vi "example test.vi"() -> ()   [LabVIEW 2014, in "alarms module tests.lvlib"]
uses:
  alarms module tests.lvlib
  module/configuration/alarms module configuration.lvclass
  module/execution/alarms module runtime.lvclass
  module/configuration/alarm configuration.ctl
  module/configuration/alarm comparison.ctl
  <vilib>/NI/Tag Bus Module Framework/channel/TBM channel.lvclass
  module/configuration/compare type.ctl
  module/configuration/boolean operation.ctl
  <vilib>/NI/Tag Bus/tag/Data Type.ctl
  <vilib>/NI/Tag Bus Module Framework/channel/channel classification.ctl
  module/configuration/alarms module configuration.lvclass/alarms module configuration.ctl
  <vilib>/NI/Tag Bus/tag/tag descriptor.lvclass/tag descriptor.ctl
  <vilib>/NI/Tag Bus/table/data polymorphs/write one/write Boolean.vi
  <vilib>/NI/Tag Bus/table/data polymorphs/write one/write Double.vi
  <vilib>/NI/Tag Bus/table/data polymorphs/write one/write U64.vi
  <vilib>/NI/Tag Bus/table/data polymorphs/read one/read Boolean.vi
  module/configuration/Write alarms.vi
  <vilib>/NI/Tag Bus/tag/read tag name.vi
  <vilib>/NI/Tag Bus/dictionary/locate tag.vi
  <vilib>/NI/Configuration Framework/serializable configuration/NISE_CEF_serializable configuration.lvclass
  <vilib>/NI/Tag Bus/tag/tag descriptor.lvclass
  <vilib>/NI/Tag Bus/dictionary/data dictionary.lvclass
  <vilib>/NI/Tag Bus/table/data table.lvlib
panel:
  in  "a":dbl
  in  "b":u64
  in  "unlatch":bool
  in  "stop":bool
  out "out":bool
  out "final error":errorcluster
  out "output error":errorcluster
  out "input lookup error":errorcluster
  out "init error":errorcluster
  out "correct execution settings":bool
  out "serialization problem":errorcluster
  out "invalid configuration":errorcluster
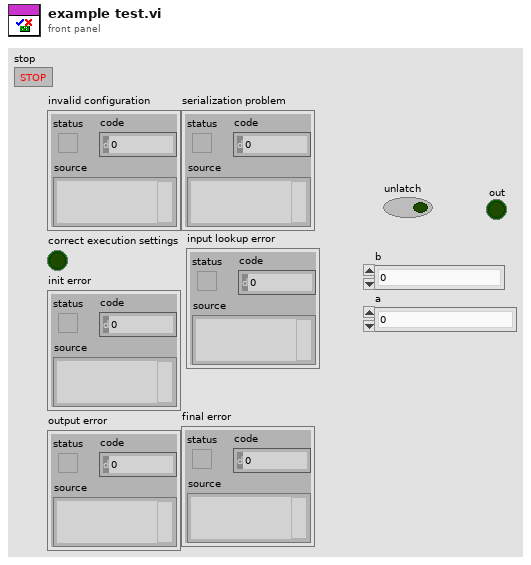
[diagram p1: front panel]
types:
  T1 = typedef "TBM channel.lvclass/channel classification.ctl" = enum16{"input data", "output data", "processing parameter", "processing result"}
  T2 = typedef "tag bus.lvlib/tag descriptor.lvclass/Data Type.ctl" = enum16{"Double", "Single", "I64", "I32", "I16", "I8", "U64", "U32", "U16", "U8", "Boolean", "String", "Array of Double", "Array of Single", "Array of I64", "Array of I32", "Array of I16", "Array of I8", "Array of U64", "Array of U32", "Array of U16", "Array of U8", "Array of Boolean", "Array of String"}
  T3 = typedef "alarms module configuration.lvclass/compare type.ctl" = enum16{">", "<", ">=", "<=", "="}
  T4 = typedef "alarms module configuration.lvclass/boolean operation.ctl" = enum16{"AND", "OR"}
  T5 = typedef "alarms module configuration.lvclass/alarm comparison.ctl" = cluster{"input channel":refnum<class "TBM channel.lvclass">, "limit":dbl, "comparison":T3}
  T6 = typedef "alarms module configuration.lvclass/alarm configuration.ctl" = cluster{"comparison":string, "comparisons":T5[], "unlatch":refnum<class "TBM channel.lvclass">, "output":refnum<class "TBM channel.lvclass">, "boolean op":T4}
  T7 = typedef "TBM channel.lvclass/data tables.ctl" = cluster{"input data":T8, "processing parameter":T8, "processing result":T8, "output data":T8}
  T8 = typedef "tag bus.lvlib/dictionary table pair.ctl" = cluster{"data dictionary":refnum<class "data dictionary.lvclass">, "data table":T9}
  T9 = typedef "tag bus.lvlib/data table.lvlib/data table.ctl" = cluster{"Double":dbl[], "Single":sgl[], "I64":i64[], "I32":i32[], "I16":i16[], "I8":i8[], "U64":u64[], "U32":u32[], "U16":u16[], "U8":u8[], "Boolean":bool[], "String":string[], "Array of Double":cluster{"DBL Array":dbl[]}[], "Array of Single":cluster{"SGL Array":sgl[]}[], "Array of I64":cluster{"I64 Array":i64[]}[], "Array of I32":cluster{"I32 Array":i32[]}[], "Array of I16":cluster{"I16 Array":i16[]}[], "Array of I8":cluster{"I8 Array":i8[]}[], "Array of U64":cluster{"U64 Array":u64[]}[], "Array of U32":cluster{"U32 Array":u32[]}[], "Array of U16":cluster{"U16 Array":u16[]}[], "Array of U8":cluster{"U8 Array":u8[]}[], "Array of Boolean":cluster{"Boolean Array":bool[]}[], "Array of String":cluster{"String Array":string[]}[]}
  T10 = typedef "TBM module execution interface.lvclass/execution settings.ctl" = cluster{"reads inputs":bool, "processes data":bool, "writes outputs":bool, "background daemon":bool}
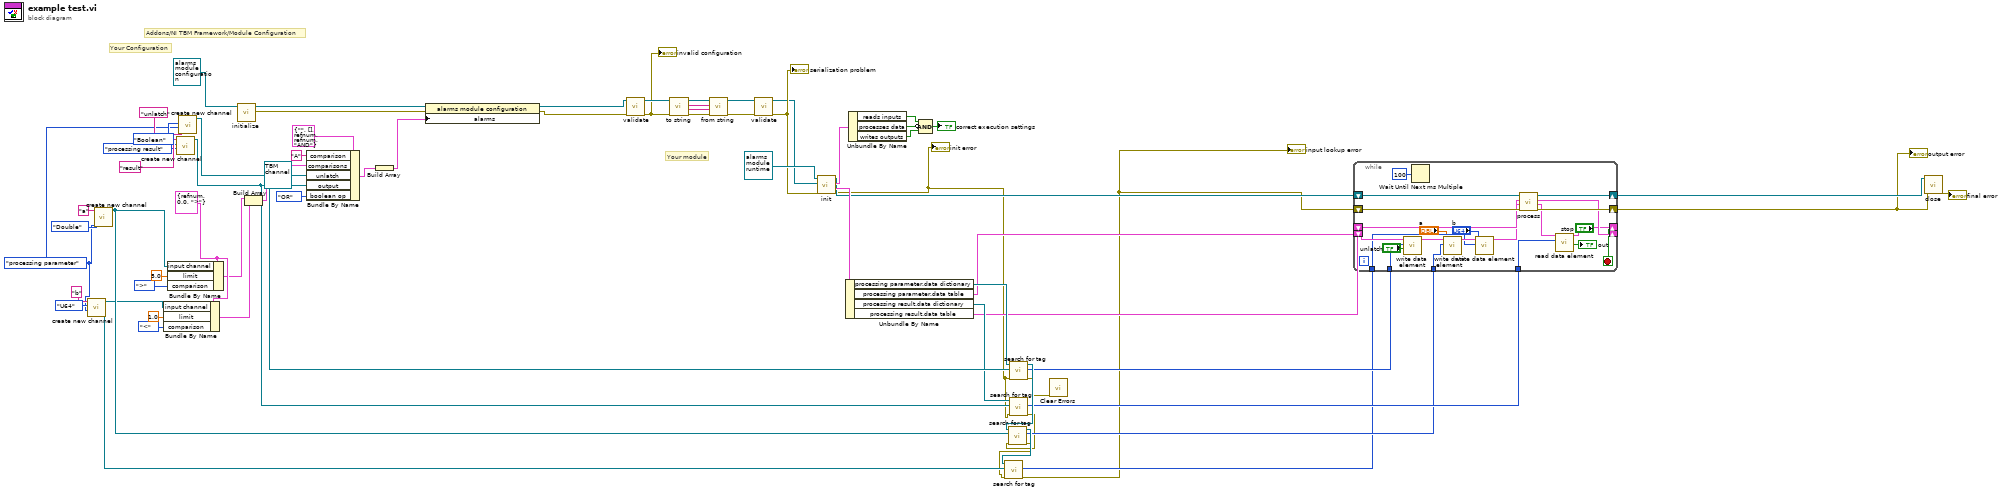
[diagram p0: block diagram]
diagram:
  w24 = channel_classification."processing parameter" ("channel classification")
  w34 = Data_Type."Boolean" ("data type")
  w42 = T5 {"input channel"=refnum, "limit"=0.0, "comparison"=enum.">"} ("alarm cfg")
  # "Your module"
  # "Your Configuration"
  # "Addons/NI TBM Framework/Module Configuration"
  n1 = call <vilib>:"create new channel.vi"("channel classification"=w24, "data type"=Data_Type."U64", "channel name"="b") -> ("channel"=w17:refnum<class "TBM channel.lvclass">)  [unwired: 8 in]
  n2 = call <vilib>:"create new channel.vi"("channel classification"=w24, "data type"=Data_Type."Double", "channel name"="a") -> ("channel"=w18:refnum<class "TBM channel.lvclass">)  [unwired: 8 in]
  n3 = Bundle By Name(cluster=w42, "input channel"=w17, "limit"=1.0, "comparison"=compare_type."<") -> (w40:T5)
  n4 = Bundle By Name(cluster=w42, "input channel"=w18, "limit"=5.0, "comparison"=compare_type.">") -> (w41:T5)
  n5 = call <vilib>:"create new channel.vi"("channel classification"=channel_classification."processing result", "data type"=w34, "channel name"="result") -> ("channel"=w19:refnum<class "TBM channel.lvclass">)  [unwired: 8 in]
  n6 = call <vilib>:"create new channel.vi"("channel classification"=w24, "data type"=w34, "channel name"="unlatch") -> ("channel"=w20:refnum<class "TBM channel.lvclass">)  [unwired: 8 in]
  n7 = call <vilib>:"initialize.vi"("configuration in"=refnum<class "alarms module configuration.lvclass"> refnum ("tag bus configurable plugin module configuration")) -> ("error out"=w49:errorcluster, "configuration out"=w48:refnum<class "alarms module configuration.lvclass">)  [unwired: 8 in, 1 out]
  n8 = Build Array(w41, w40) -> (w39:T5[])
  n9 = Bundle By Name(cluster=T6 {"comparison"="", "comparisons"=[], "unlatch"=refnum, "output"=refnum, "boolean op"=enum."AND"} ("alarm config"), "comparison"="A", "comparisons"=w39, "unlatch"=refnum<class "TBM channel.lvclass"> refnum, "output"=w19, "boolean op"=boolean_operation."OR") -> (w44:T6)
  n10 = Build Array(w44) -> (w43:T6[])
  n11 = property class="alarms module configuration"(reference=w48, error in=w49, "alarms"=w43) -> (reference out=w46:refnum<class "alarms module configuration.lvclass">, error out=w47:errorcluster)
  n12 = call-dynamic "validate.vi"("error in"=w47, "alarms module configuration in"=w46) -> ("error out"=w67:errorcluster, "alarms module configuration out"=w68:refnum<class "alarms module configuration.lvclass">)  [unwired: 8 in]
  "invalid configuration" <- w67
  n13 = call-dynamic "to string.vi"("error in"=w67, "alarms module configuration in"=w68) -> ("error out"=w63:errorcluster, "data"=w64:string, "version"=w65:string, "alarms module configuration out"=w66:refnum<class "alarms module configuration.lvclass">)  [unwired: 6 in]
  n14 = call-dynamic "from string.vi"("error in"=w63, "data"=w64, "version"=w65, "alarms module configuration in"=w66) -> ("error out"=w61:errorcluster, "alarms module configuration out"=w62:refnum<class "alarms module configuration.lvclass">)  [unwired: 6 in]
  n15 = call-dynamic "validate.vi"("error in"=w61, "alarms module configuration in"=w62) -> ("error out"=w59:errorcluster, "alarms module configuration out"=w58:refnum<class "alarms module configuration.lvclass">)  [unwired: 8 in]
  "serialization problem" <- w59
  n16 = call-dynamic "init.vi"("error in"=w59, "TBM module configuration in"=w58, "alarms module runtime in"=refnum<class "alarms module runtime.lvclass"> refnum ("tag bus configurable plugin module")) -> ("error out"=w2:errorcluster, "data allocations"=w52:T7, "execution settings"=w57:T10, "alarms module runtime out"=w23:refnum<class "alarms module runtime.lvclass">)  [unwired: 5 in]
  "init error" <- w2
  n17 = Unbundle By Name(w52) -> ("processing parameter.data dictionary"=w16:refnum<class "data dictionary.lvclass">, "processing parameter.data table"=w12:T9, "processing result.data dictionary"=w13:refnum<class "data dictionary.lvclass">, "processing result.data table"=w11:T9)
  n18 = Unbundle By Name(w57) -> ("reads inputs"=w54:bool, "processes data"=w56:bool, "writes outputs"=w55:bool)
  n19 = Compound Arithmetic op=AND(w54, invert w56, w55) -> (→"correct execution settings":bool)
  n20 = call <vilib>:"search for tag.vi"("error in"=w2, "system tag"=w20, "data dictionary in"=w16) -> ("error out"=w1:errorcluster, "index"=w9:i32, "data dictionary out"=w15:refnum<class "data dictionary.lvclass">)  [unwired: 6 in]
  n21 = call <vilib>:"search for tag.vi"("error in"=w2, "system tag"=w19, "data dictionary in"=w13) -> ("error out"=w6:errorcluster, "index"=w10:i32)  [unwired: 6 in, 1 out]
  n22 = call <vilib>:"search for tag.vi"("error in"=w6, "system tag"=w18, "data dictionary in"=w15) -> ("error out"=w5:errorcluster, "index"=w8:i32, "data dictionary out"=w14:refnum<class "data dictionary.lvclass">)  [unwired: 6 in]
  n23 = call <vilib>:"search for tag.vi"("error in"=w5, "system tag"=w17, "data dictionary in"=w14) -> ("error out"=w4:errorcluster, "index"=w7:i32)  [unwired: 6 in, 1 out]
  "input lookup error" <- w4
  n24 = call <vilib>:"Clear Errors.vi"("error in (no error)"=w1) -> ()  [unwired: 5 in, 2 out]
  n25 = while {
    shift-right: [w89] -> w22
    shift-left: w23 -> [w90]
    shift-right: [w87] -> w21
    shift-left: w4 -> [w88]
    shift-right: [w86] -> _
    shift-left: w12 -> [w82]
    shift-right: [w79] -> _
    shift-left: w11 -> [w85]
    tunnel: w10 -> [w78]
    tunnel: w9 -> [w74]
    tunnel: w8 -> [w72]
    tunnel: w7 -> [w71]
    stop <- "stop" stop-if-true
    n26 = call-poly <vilib>:"write data element.vi"("value"="unlatch", "index"=w74, "data table in"=w82) -> ("data table out"=w83:T9)  [unwired: 8 in]
    n27 = Wait Until Next ms Multiple(millisecond multiple=u32 100) -> ()  [unwired: 1 out]
    n28 = call-poly <vilib>:"write data element.vi"("value"="a", "index"=w72, "data table in"=w83) -> ("data table out"=w84:T9)  [unwired: 8 in]
    n29 = call-poly <vilib>:"write data element.vi"("value"="b", "index"=w71, "data table in"=w84) -> ("data table out"=w81:T9)  [unwired: 8 in]
    n30 = call-dynamic "process.vi"("error in"=w88, "result allocation"=w85, "parameters"=w81, "module in"=w90) -> ("error out"=w87:errorcluster, "results"=w80:T9, "parameter allocation"=w86:T9, "module out"=w89:refnum<class "alarms module runtime.lvclass">)  [unwired: 4 in]
    n31 = call-poly <vilib>:"read data element.vi"("index"=w78, "data table in"=w80) -> ("value"=→"out":bool, "data table out"=w79:T9)  [unwired: 8 in]
  }
  "output error" <- w21
  n32 = call-dynamic "close.vi"("error in"=w21, "alarms module runtime in"=w22) -> ("error out"=→"final error":errorcluster)  [unwired: 9 in]
